vi "Visual - Index Data_SubVIs-某型振动实验台测试系统.vi"(8 "Error In":errorcluster, 11 "Data":dbl[][](array[numeric])) -> (0 "Error Out":errorcluster, 3 "Data":waveform(dbl)[](array[waveform]))   [LabVIEW 2009]
doc: "Use this template to build a VI to use as a subVI."
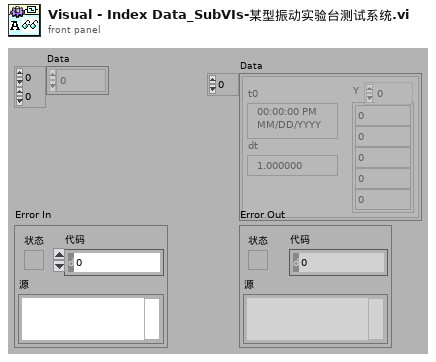
[diagram p1: front panel]
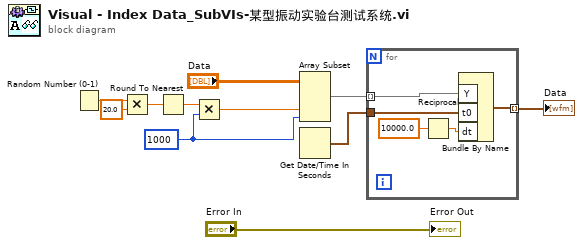
[diagram p0: block diagram]
diagram:
  w1 = 1000 ("length")
  n1 = Random Number (0-1)() -> (number: 0 to 1=w10:dbl)
  n2 = Multiply(x=w10, y=20.0) -> (x*y=w4:dbl)
  n3 = Round To Nearest(number=w4) -> (nearest integer value=w3:dbl)
  n4 = Multiply(x=w3, y=w1) -> (x*y=w2:dbl)
  n5 = Array Subset(array="Data", index (col)=w2, length (col)=w1) -> (w7:dbl[][])  [unwired: 2 in]
  n6 = Get Date/Time In Seconds() -> (seconds since 1Jan1904=w6:timestamp)
  n7 = for {
    tunnel: w7 -> [w16] mode=indexing
    tunnel: w6 -> [w15]
    tunnel: [w12] -> w5 mode=indexing
    n8 = Reciprocal(x=10000.0 ("dt")) -> (1/x=w13:dbl)
    n9 = Bundle By Name("Y"=w16, "t0"=w15, "dt"=w13) -> (w12:waveform(dbl))  [unwired: 1 out]
  }
  "Data" <- w5
  "Error Out" <- "Error In"
